vi "Block Average.vi"(9 "Subset Length":i32, 11 "Input Array":dbl[][](array[numeric])) -> (3 "Block Averaged Array":dbl[][](array[numeric]))   [LabVIEW 2018]
uses:
  <vilib>/Analysis/baseanly.llb/Mean (DBL).vi
  <vilib>/Analysis/NI_AALBase.lvlib
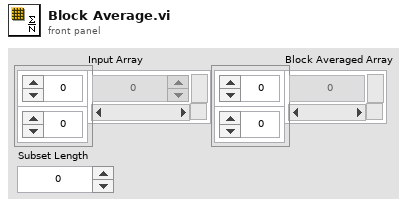
[diagram p1: front panel]
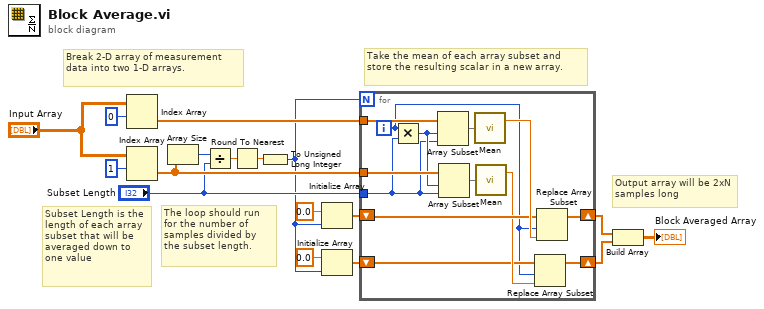
[diagram p0: block diagram]
diagram:
  # "Take the mean of each array subset and store the resulting scalar in a new array."
  # "Output array will be 2xN samples long"
  # "The loop should run for the number of samples divided by the subset length."
  # "Subset Length is the length of each array subset that will be averaged down to one value"
  # "Break 2-D array of measurement data into two 1-D arrays."
  n1 = Index Array(array="Input Array", index (row)=0) -> (element=w15:dbl[])  [unwired: 1 in]
  n2 = Index Array(array="Input Array", index (row)=1) -> (element=w5:dbl[])  [unwired: 1 in]
  n3 = Array Size(array=w5) -> (size(s)=w6:i32)
  n4 = Divide(x=w6, y="Subset Length") -> (x/y=w3:dbl)
  n5 = Round To Nearest(number=w3) -> (nearest integer value=w2:dbl)
  n6 = To Unsigned Long Integer(number=w2) -> (unsigned 32bit integer=w1:u32)
  n7 = Initialize Array(0.0, w1) -> (w13:dbl[])
  n8 = Initialize Array(0.0, w1) -> (w11:dbl[])
  n9 = for {
    N: w1 -> [_]
    tunnel: w15 -> [w30]
    tunnel: "Subset Length" -> [w25]
    shift-right: [w18] -> w10
    shift-left: w13 -> [w23]
    shift-right: [w19] -> w9
    shift-left: w11 -> [w21]
    tunnel: w5 -> [w28]
    i -> [w20]
    n10 = Multiply(x=w20, y=w25) -> (x*y=w26:i32)
    n11 = Array Subset(array=w30, index=w26, length=w25) -> (w29:dbl[])
    n12 = Array Subset(array=w28, index=w26, length=w25) -> (w27:dbl[])
    n13 = call-poly <vilib>:"Mean.vi"("X"=w29) -> ("mean"=w24:dbl)  [unwired: 1 out]
    n14 = call-poly <vilib>:"Mean.vi"("X"=w27) -> ("mean"=w22:dbl)  [unwired: 1 out]
    n15 = Replace Array Subset(array=w21, new element=w22, index=w20) -> (w19:dbl[])
    n16 = Replace Array Subset(array=w23, new element=w24, index=w20) -> (w18:dbl[])
  }
  n17 = Build Array(w10, w9) -> (→"Block Averaged Array":dbl[][])
